vi "Ref.vi"(11 "GUI Element in":refnum<class "GUI Element.lvclass">) -> (2 "Ref":refnum<vi>, 3 "GUI Element out":refnum<class "GUI Element.lvclass">)   [LabVIEW 2020, in "VolatusGUI.lvlib" / "GUI Element.lvclass"]
uses:
  GUI Element.lvclass
  GUI Element.lvclass/GUI Element.ctl
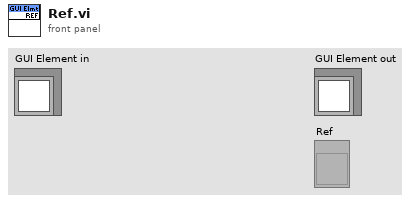
[diagram p1: front panel]
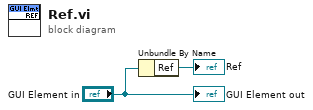
[diagram p0: block diagram]
diagram:
  n1 = Unbundle By Name("GUI Element in") -> ("Ref"=→"Ref":refnum<vi>)
  "GUI Element out" <- "GUI Element in"
